vi "Streamline2003.vi"   [LabVIEW 2013]
uses:
  <vilib>/Heliosphere Research LLC/Advanced Plotting Toolkit/Advanced Plotting Toolkit.lvlib
types:
  T1 = typedef "Advanced Plotting Toolkit.lvlib/PlotID.ctl" = i32
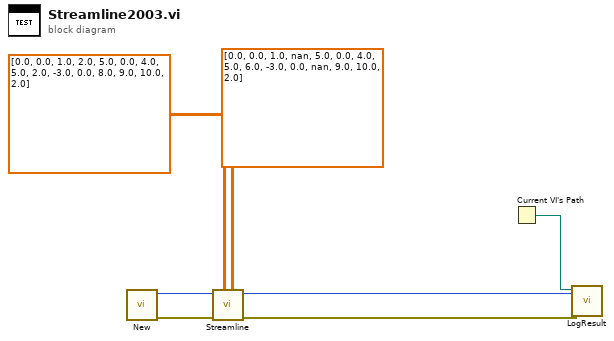
[diagram p0: block diagram]
diagram:
  n1 = call <vilib>:"New.vi"() -> ("error out"=w5:errorcluster, "Plot ID"=w6:T1)  [unwired: 10 in]
  n2 = call <vilib>:"Streamline.vi"("Y Vector Component"=dbl[][] [[0.0, 0.0, 1.0, nan, 5.0], [0.0, 4.0, 5.0, 6.0, -3.0], [0.0, nan, 9.0, 10.0, 2.0]] ("Data"), "X Vector Component"=dbl[][] [[0.0, 0.0, 1.0, 2.0, 5.0], [0.0, 4.0, 5.0, 2.0, -3.0], [0.0, 8.0, 9.0, 10.0, 2.0]] ("Data"), "error in (no error)"=w5, "Plot ID"=w6) -> ("error out"=w3:errorcluster, "Plot ID Out"=w4:T1)  [unwired: 6 in]
  n3 = Current VI's Path() -> (path=w7:path)
  n4 = call "LogResult.vi"("Test Result"=w3, "Test Artifact"=w4, "VI Path"=w7) -> ()  [unwired: 9 in]
